vi "UtilityLib.remove white spaces.vi"(0 "string with blanks":string) -> (14 "string without white spaces":string, 15 "whiteSpacesRemovedFront":string, 16 "nRemovedFront":i32, 17 "whiteSpacesRemovedBack":string, 18 "nRemovedBack":i32)   [LabVIEW 2015, in "UtilityLib.lvlib"]
doc: "Removes any white spaces (tabs, carriage returns, blanks, \\00 and linefeeds) from the beginning and the end of a string. The main idea behind this VI was to return the number of white spaces and the removed white spaces as well."
uses:
  UtilityLib.lvlib
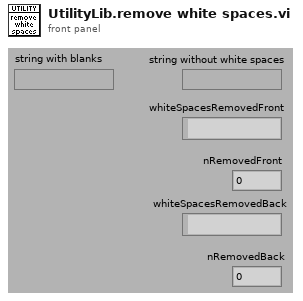
[diagram p1: front panel]
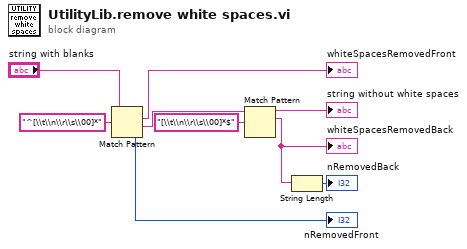
[diagram p0: block diagram]
diagram:
  n1 = Match Pattern(string="string with blanks", regular expression="^[\\t\\n\\r\\s\\00]*") -> (match substring=→"whiteSpacesRemovedFront":string, after substring=w8:string, offset past match=→"nRemovedFront":i32)  [unwired: 1 in, 1 out]
  n2 = Match Pattern(string=w8, regular expression="[\\t\\n\\r\\s\\00]*$") -> (before substring=→"string without white spaces":string, match substring=w4:string)  [unwired: 1 in, 2 out]
  "whiteSpacesRemovedBack" <- w4
  n3 = String Length(string=w4) -> (length=→"nRemovedBack":i32)
